vi "Parse Tag.vi"(8 "Error In":errorcluster, 11 "Parser In":refnum<class "Parser.lvclass">) -> (0 "Error Out":errorcluster, 2 "End?":bool, 3 "Parser Out":refnum<class "Parser.lvclass">)   [LabVIEW 2017, in "Mustache.lvlib" / "Parser.lvclass"]
uses:
  Parser.lvclass
  Public/Controls/States.ctl
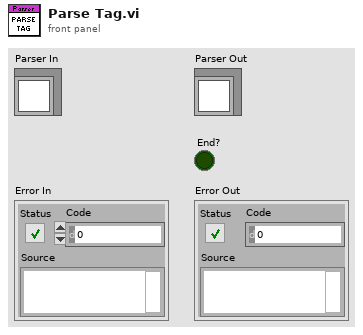
[diagram p1: front panel]
types:
  T1 = typedef "Mustache.lvlib/Parser.lvclass/States.ctl" = enum16{"Text", "Opening Tag", "Tag", "Closing Tag"}
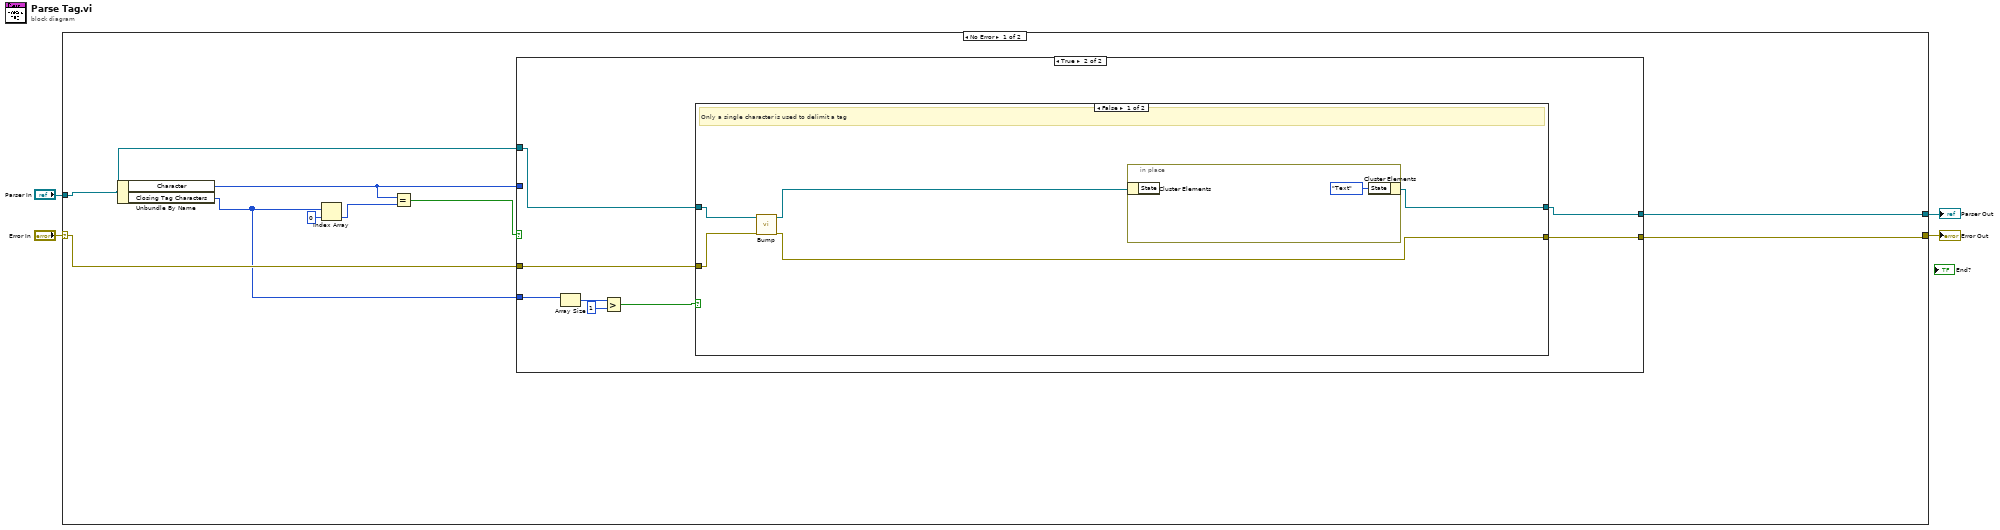
[diagram p0: block diagram]
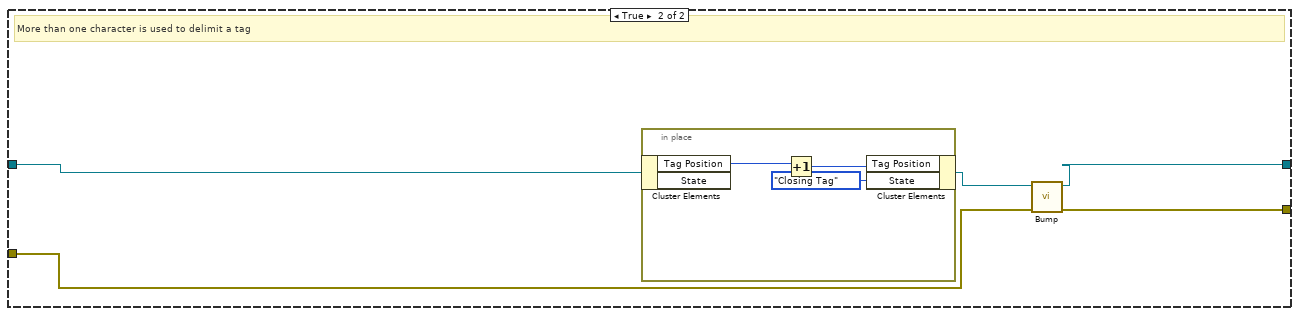
[diagram p3: hidden frame]
diagram:
  n1 = case shown="No Error" "Error In" {
    selector: "Error In" -> [w12 w36]
    tunnel: [w5 w36] -> w4
    tunnel: [w6 w37] -> w3
    tunnel: "Parser In" -> [w13 w37]
    frame No Error {
      n2 = Unbundle By Name(w13) -> ("Character"=w10:u8, "Closing Tag Characters"=w7:u8[])
      n3 = Index Array(array=w7, index=0) -> (element=w9:u8)
      n4 = Equal?(x=w10, y=w9) -> (x = y?=w8:bool)
      n5 = case shown="True" w8 {
        tunnel: w13 -> [_ w17]
        tunnel: w12 -> [_ w15]
        tunnel: w10 -> [_ _]
        tunnel: w7 -> [_ w21]
        tunnel: [_ w16] -> w6
        tunnel: [_ w14] -> w5
        frame False {
        }
        frame True {
          n6 = Array Size(array=w21) -> (size(s)=w20:i32)
          n7 = Greater?(x=w20, y=1) -> (0:w18:bool)
          n8 = case shown="False" w18 {
            tunnel: w17 -> [w25 w32]
            tunnel: [w26 w30] -> w16
            tunnel: w15 -> [w23 w29]
            tunnel: [w22 w28] -> w14
            frame False {
              # "Only a single character is used to delimit a tag"
              n9 = call "Bump.vi"("Error In"=w23, "Parser In"=w25) -> ("Error Out"=w22:errorcluster, "Parser Out"=w24:refnum<class "Parser.lvclass">)  [unwired: 8 in]
              n10 = in-place {
                n11 = in-place-cluster #1(w24) -> ()  [unwired: 1 out]
                n12 = in-place-cluster #1("State"=States."Text") -> (w26:refnum<class "Parser.lvclass">)
              }
            }
            frame True {
              # "More than one character is used to delimit a tag"
              n13 = in-place {
                n14 = in-place-cluster #2(w32) -> ("Tag Position"=w35:i32)  [unwired: 1 out]
                n15 = Increment(x=w35) -> (x+1=w34:i32)
                n16 = in-place-cluster #2("Tag Position"=w34, "State"=States."Closing Tag") -> (w31:refnum<class "Parser.lvclass">)
              }
              n17 = call "Bump.vi"("Error In"=w29, "Parser In"=w31) -> ("Error Out"=w28:errorcluster, "Parser Out"=w30:refnum<class "Parser.lvclass">)  [unwired: 8 in]
            }
          }
        }
      }
    }
    frame Error {
    }
  }
  "Error Out" <- w4
  "Parser Out" <- w3
